vi "AssertXPathConnectorPanesMatchTemplateFiles.vi"(6 "terminal subset acceptable (false)":bool, 8 "error in (no error)":errorcluster, 9 "absolute custom device xml file":path, 10 "connector pane templates":T1[](array[typedef]), 11 "TestCase in":refnum<class "TestCase.lvclass">) -> (0 "error out":errorcluster, 3 "TestCase out":refnum<class "TestCase.lvclass">)   [LabVIEW 2015, in "VeriStandTestUtilities.lvlib"]
uses:
  VeriStandTestUtilities.lvlib
  <vilib>/addons/_JKI Toolkits/VI Tester/TestCase.llb/TestCase.lvclass
  ConnectorPaneTemplate.ctl
  <vilib>/xml/Load XML File.vi
  <userlib>/_OpenG.lib/array/array.llb/Remove Duplicates from 1D Array (String)__ogtk.vi
  <vilib>/xml/Close Reference(Node).vi
  <vilib>/xml/NI_XML.lvlib
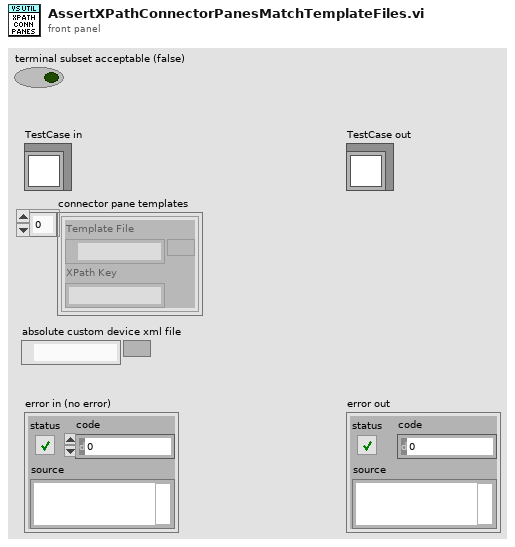
[diagram p1: front panel]
types:
  T1 = typedef "VeriStandTestUtilities.lvlib/ConnectorPaneTemplate.ctl" = cluster{"Template File":path, "XPath Key":string}
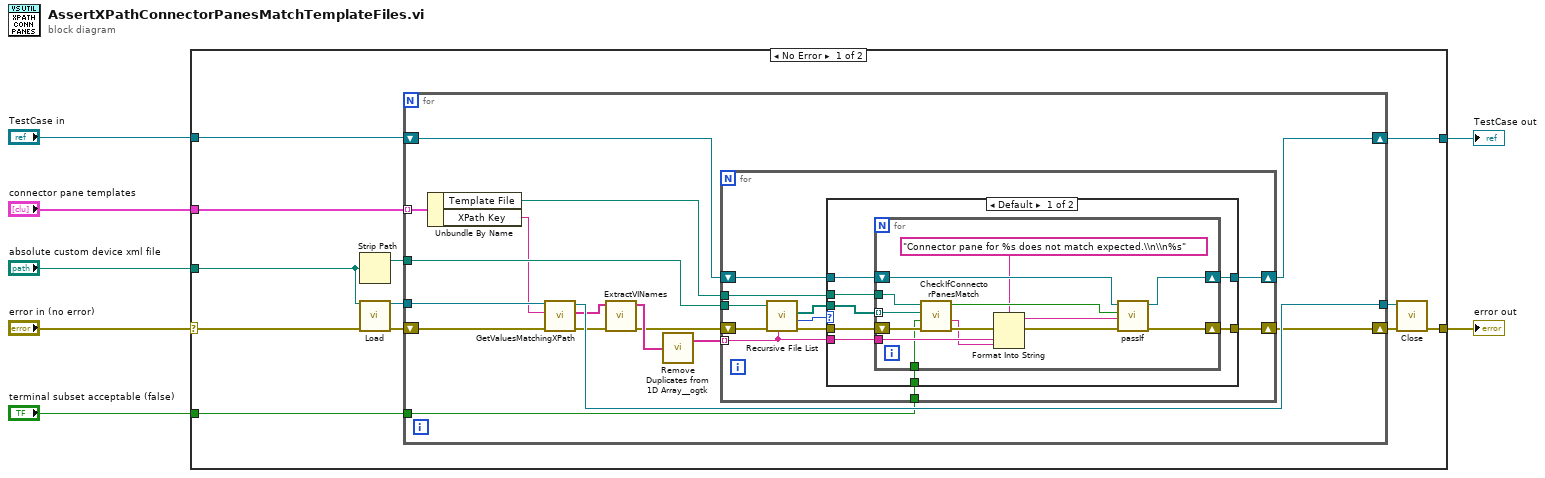
[diagram p0: block diagram]
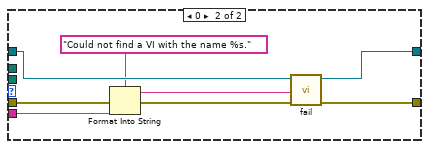
[diagram p2: hidden frame]
diagram:
  n1 = case shown="No Error" "error in (no error)" {
    selector: "error in (no error)" -> [w10 w78]
    tunnel: "absolute custom device xml file" -> [w18 _]
    tunnel: [w17 w77] -> w6
    tunnel: "TestCase in" -> [w15 w77]
    tunnel: [w13 w78] -> w4
    tunnel: "connector pane templates" -> [w9 _]
    tunnel: "terminal subset acceptable (false)" -> [w8 _]
    frame No Error {
      n2 = Strip Path(path=w18) -> (stripped path=w19:path)  [unwired: 1 out]
      n3 = call-poly <vilib>:"Load.vi"("path to XML document"=w18, "error in (no error)"=w10) -> ("DOM document out"=w12:refnum<k20>, "error out"=w11:errorcluster)  [unwired: 11 in, 1 out]
      n4 = for {
        shift-right: [w29] -> w16
        shift-left: w11 -> [w34]
        tunnel: w12 -> [w35]
        tunnel: [w33] -> w14
        tunnel: w9 -> [w27] mode=indexing
        shift-right: [w32] -> w17
        shift-left: w15 -> [w31]
        tunnel: w19 -> [w30]
        tunnel: w8 -> [w24]
        n5 = Unbundle By Name(w27) -> ("Template File"=w25:path, "XPath Key"=w26:string)
        n6 = call "GetValuesMatchingXPath.vi"("error in (no error)"=w34, "XPath"=w26, "XML refnum in"=w35) -> ("error out"=w21:errorcluster, "Values"=w23:string[], "XML refnum out"=w33:refnum<k20>)  [unwired: 6 in]
        n7 = call "ExtractVINames.vi"("error in (no error)"=w21, "vi paths"=w23) -> ("error out"=w20:errorcluster, "vi names"=w22:string[])  [unwired: 8 in]
        n8 = call-poly <userlib>:"Remove Duplicates from 1D Array__ogtk.vi"("Input Array"=w22) -> ("Output Array"=w28:string[])  [unwired: 1 out]
        n9 = for {
          shift-right: [w44] -> w29
          shift-left: w20 -> [w46]
          tunnel: w28 -> [w40] mode=indexing
          tunnel: w30 -> [w45]
          tunnel: w25 -> [w43]
          shift-right: [w41] -> w32
          shift-left: w31 -> [w42]
          tunnel: w24 -> [w36]
          n10 = call <vilib>:"Recursive File List.vi"("pattern"=w40, "error in (no error)"=w46, "Folder Path"=w45) -> ("error out"=w38:errorcluster, "Number of Files"=w39:i32, "All Files in Dir"=w37:path[])  [unwired: 4 in, 2 out]
          n11 = case shown="Default" w39 {
            tunnel: w38 -> [w54 w72]
            tunnel: [w52 w76] -> w44
            tunnel: w37 -> [w49 _]
            tunnel: w43 -> [w53 _]
            tunnel: w42 -> [w51 w75]
            tunnel: [w50 w74] -> w41
            tunnel: w40 -> [w48 w73]
            tunnel: w36 -> [w47 _]
            frame Default {
              n12 = for {
                tunnel: w53 -> [w67]
                shift-right: [w65] -> w52
                shift-left: w54 -> [w68]
                shift-right: [w63] -> w50
                shift-left: w51 -> [w64]
                tunnel: w49 -> [w62] mode=indexing
                tunnel: w48 -> [w60]
                tunnel: w47 -> [w55]
                n13 = call "CheckIfConnectorPanesMatch.vi"("error in (no error)"=w68, "terminal subset acceptable (false)"=w55, "actual connector pane vi"=w62, "expected connector pane vi"=w67) -> ("error out"=w58:errorcluster, "mismatch explanation"=w56:string, "connector panes match"=w66:bool)  [unwired: 5 in]
                n14 = Format Into String(format string="Connector pane for %s does not match expected.\\n\\n%s" ("connector pane mismatch error"), error in=w58, w60, w56) -> (resulting string=w59:string, error out=w61:errorcluster)  [unwired: 1 in]
                n15 = call-dynamic "passIf.vi"("error in (no error)"=w61, "message (\"\")"=w59, "pass"=w66, "TestCase in"=w64) -> ("error out"=w65:errorcluster, "TestCase out"=w63:refnum<class "TestCase.lvclass">)  [unwired: 6 in]
              }
            }
            frame 0 {
              n16 = Format Into String(format string="Could not find a VI with the name %s." ("no matches error"), error in=w72, w73) -> (resulting string=w70:string, error out=w71:errorcluster)  [unwired: 1 in]
              n17 = call-dynamic "fail.vi"("error in (no error)"=w71, "message (\"\")"=w70, "TestCase in"=w75) -> ("error out"=w76:errorcluster, "TestCase out"=w74:refnum<class "TestCase.lvclass">)  [unwired: 7 in]
            }
          }
        }
      }
      n18 = call-poly <vilib>:"Close.vi"("error in (no error)"=w16, "node"=w14) -> ("error out"=w13:errorcluster)  [unwired: 7 in]
    }
    frame Error {
    }
  }
  "TestCase out" <- w6
  "error out" <- w4
